vi "ALTS-2015 Add or Remove Serial Task.vi"(8 "Error in":errorcluster) -> (0 "Error Out":errorcluster)   [LabVIEW 2013]
uses:
  Controls/ALTS-2015 Serial Task Handler FGV-Command.ctl
  Controls/ALTS-2015 Serial Task Handler FGV-Operation.ctl
  Controls/ALTS-2015 Robot FIFO Queue Options.ctl
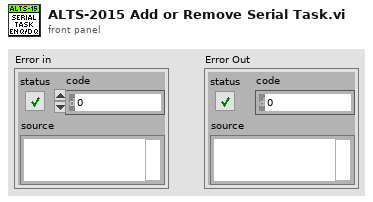
[diagram p1: front panel]
types:
  T1 = typedef "ALTS-2015 Serial Task Handler FGV-Operation.ctl" = enum16{"Replace/Insert", "No Operation"}
  T2 = typedef "ALTS-2015 Serial Task Handler FGV-Command.ctl" = enum16{"Set Replace/Insert Falg", "Get Status", "Reset Flag", "Reset S Data"}
  T3 = typedef "ALTS-2015 Robot FIFO Queue Options.ctl" = enum16{"Init", "Enqueue", "Dequeue", "Get Queue Elements", "Flush", "Destroy"}
  T4 = typedef "ALTS-2015 Serial Details.ctl" = cluster{"Robot Task":T5, "Serial No":string, "New Serial?":bool, "Station # Unload":T6, "Last Test Result":bool, "Rerun?":bool, "Station # Rerun":T6, "Invalid Serial?":bool, "Serial Details":T7}
  T5 = typedef "ALTS-2015 Robot Tasks.ctl" = enum16{"Load", "Unload", "Rerun", "Invalid Serial"}
  T6 = typedef "ALTS-2015 Station Cluster.ctl" = enum16{"Station 1", "Station 2", "Station 3", "Station 4"}
  T7 = typedef "ALTS-2015 Serial DB Details.ctl" = cluster{"Adapter Plate Size":i32, "Air Leak Test Type ":i32, "Displacement Size":i32, "Flange Size":i32, "Height":i32, "Load Decision":i32, "Cart Insert":i32}
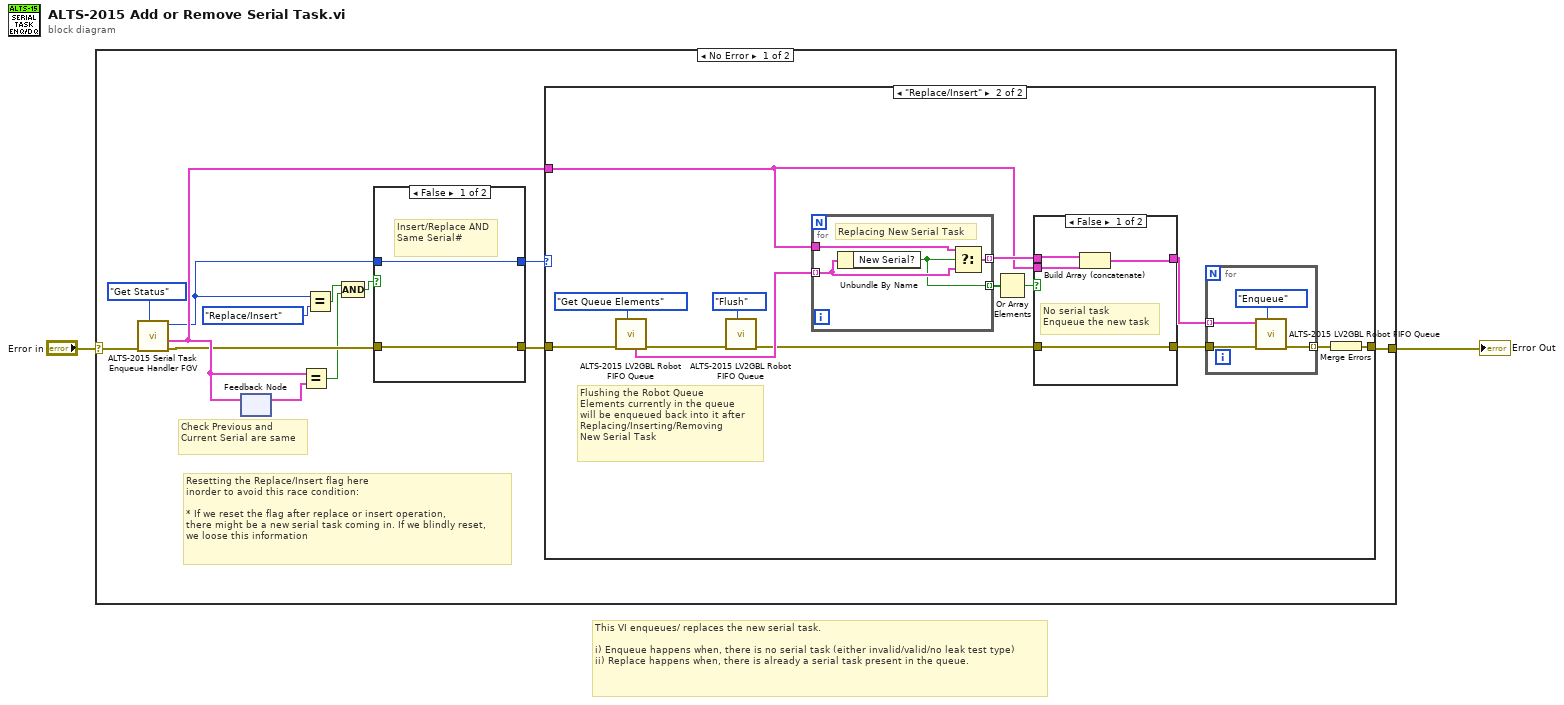
[diagram p0: block diagram]
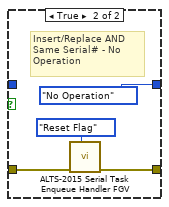
[diagram p2: hidden frame]
diagram:
  # "This VI enqueues/ replaces the new serial task. \n\ni) Enqueue happens when, there is no serial task (either invalid/valid/no leak test type)\nii) Replace happens when, there is already a serial task present in the queue."
  n1 = case shown="No Error" "Error in" {
    selector: "Error in" -> [w15 w51]
    tunnel: [w13 w51] -> w1
    frame No Error {
      # "Check Previous and Current Serial are same"
      # "Resetting the Replace/Insert flag here\ninorder to avoid this race condition:\n\n* If we reset the flag after replace or insert operation,\nthere might be a new serial task coming in. If we blindly reset,\nwe loose this information"
      n2 = call "ALTS-2015 Serial Task Enqueue Handler FGV.vi"("Command"=ALTS-2015_Serial_Task_Handler_FGV-Command."Get Status", "Error In"=w15) -> ("Error Out"=w8:errorcluster, "Task Details Out"=w11:T4, "Operation"=w10:T1)  [unwired: 7 in]
      n3 = feedback #1() -> (w12:T4)  [unwired: 1 in]
      n4 = feedback-in #1(w11) -> ()
      n5 = Equal?(x=w11, y=w12) -> (x = y?=w4:bool)
      n6 = Equal?(x=w10, y=ALTS-2015_Serial_Task_Handler_FGV-Operation."Replace/Insert") -> (x = y?=w5:bool)
      n7 = Compound Arithmetic op=AND(w5, w4) -> (w3:bool)
      n8 = case "Insert/Replace AND Same Serial#" shown="False" w3 {
        tunnel: w10 -> [w17 _]
        tunnel: [w17 ALTS-2015_Serial_Task_Handler_FGV-Operation."No Operation" ("Operation")] -> w9
        tunnel: w8 -> [w16 w21]
        tunnel: [w16 w19] -> w7
        frame False {
          # "Insert/Replace AND Same Serial#"
        }
        frame True {
          # "Insert/Replace AND Same Serial# - No Operation"
          n9 = call "ALTS-2015 Serial Task Enqueue Handler FGV.vi"("Command"=ALTS-2015_Serial_Task_Handler_FGV-Command."Reset Flag", "Error In"=w21) -> ("Error Out"=w19:errorcluster)  [unwired: 7 in, 2 out]
        }
      }
      n10 = case shown="\"Replace/Insert\"" w9 {
        tunnel: w7 -> [w22 w32]
        tunnel: [w22 w23] -> w13
        tunnel: w11 -> [_ w25]
        frame "No Operation" {
        }
        frame "Replace/Insert" {
          # "Flushing the Robot Queue\nElements currently in the queue\nwill be enqueued back into it after \nReplacing/Inserting/Removing \nNew Serial Task"
          n11 = call "ALTS-2015 LV2GBL Robot FIFO Queue.vi"("Options"=ALTS-2015_Robot_FIFO_Queue_Options."Get Queue Elements" ("Enum"), "error in (no error)"=w32) -> ("error out"=w33:errorcluster, "elements"=w36:T4[])  [unwired: 5 in, 3 out]
          n12 = call "ALTS-2015 LV2GBL Robot FIFO Queue.vi"("Options"=ALTS-2015_Robot_FIFO_Queue_Options."Flush" ("Enum"), "error in (no error)"=w33) -> ("error out"=w29:errorcluster)  [unwired: 5 in, 4 out]
          n13 = for {
            tunnel: w36 -> [w49] mode=indexing
            tunnel: [w50] -> w27 mode=indexing
            tunnel: w25 -> [w48]
            tunnel: [w47] -> w30 mode=indexing
            # "Replacing New Serial Task"
            n14 = Unbundle By Name(w49) -> ("New Serial?"=w47:bool)
            n15 = Select(t=w48, s=w47, f=w49) -> (s? t:f=w50:T4)
          }
          n16 = Or Array Elements(Boolean array=w30) -> (logical OR=w28:bool)
          n17 = case shown="False" w28 {
            tunnel: w29 -> [w37 w41]
            tunnel: w27 -> [w40 w42]
            tunnel: [w38 w42] -> w26
            tunnel: w25 -> [w39 _]
            tunnel: [w37 w41] -> w24
            frame False {
              # "No serial task\nEnqueue the new task"
              n18 = Build Array (concatenate)(w40, w39) -> (w38:T4[])
            }
            frame True {
              # "Replaced the Old task"
            }
          }
          n19 = for {
            tunnel: w24 -> [w45]
            tunnel: w26 -> [w44] mode=indexing
            tunnel: [w43] -> w31 mode=indexing
            n20 = call "ALTS-2015 LV2GBL Robot FIFO Queue.vi"("Options"=ALTS-2015_Robot_FIFO_Queue_Options."Enqueue" ("Enum"), "error in (no error)"=w45, "Task Details In"=w44) -> ("error out"=w43:errorcluster)  [unwired: 4 in, 4 out]
          }
          n21 = Merge Errors(w31) -> (w23:errorcluster)
        }
      }
    }
    frame Error {
    }
  }
  "Error Out" <- w1
